vi "GroupRelayControl.vi"(8 "error in (no error)":errorcluster, 9 "Actions":string, 10 "relay names":string, 11 "IVI Refnum in":refnum<k15>) -> (0 "error out":errorcluster, 3 "IVI Refnum out":refnum<k15>)   [LabVIEW 2015]
doc: "Use comma(,) to separate relay names\nExample\nk1,k2,k4\n\nFor action\n20 - Open Relay\n21 - Close Relay\nExample\n20,21,21"
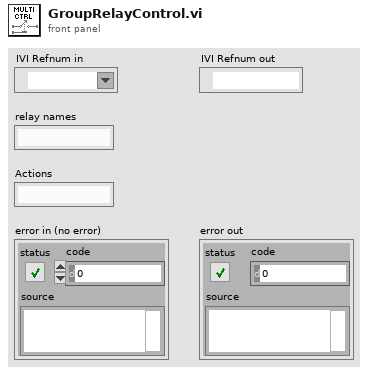
[diagram p1: front panel]
types:
  T1 = typedef "niSwitch Relay Action.ctl" = i32
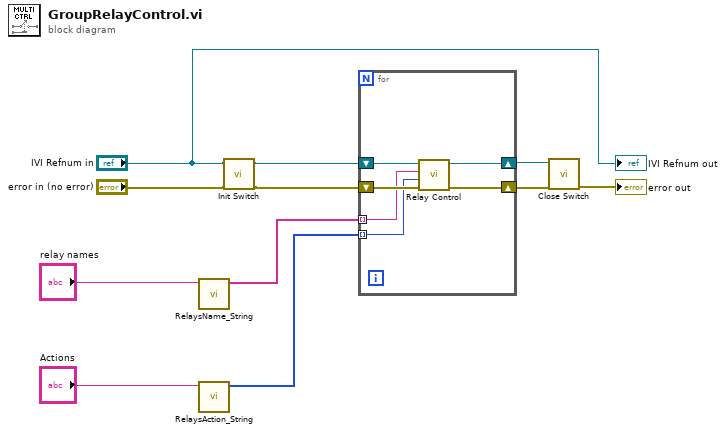
[diagram p0: block diagram]
diagram:
  n1 = call "RelaysName_String.vi"("relay names"="relay names") -> ("Array"=w10:string[])  [unwired: 10 in]
  n2 = call "RelaysAction_String.vi"("Actions"="Actions") -> ("array"=w11:T1[])  [unwired: 10 in]
  n3 = call "Init Switch.vi"("error in (no error)"="error in (no error)", "resource name"="IVI Refnum in") -> ("error out"=w4:errorcluster, "instrument handle out"=w7:refnum<k15>)  [unwired: 8 in]
  n4 = for {
    shift-right: [w15] -> w2
    shift-left: w4 -> [w17]
    shift-right: [w14] -> w3
    shift-left: w7 -> [w16]
    tunnel: w10 -> [w13] mode=indexing
    tunnel: w11 -> [w12] mode=indexing
    n5 = call "Relay Control.vi"("error in (no error)"=w17, "relay action (Close Relay)"=w12, "relay names"=w13, "instrument handle"=w16) -> ("error out"=w15:errorcluster, "instrument handle out"=w14:refnum<k15>)  [unwired: 6 in]
  }
  n6 = call "Close Switch.vi"("error in (no error)"=w2, "instrument handle"=w3) -> ("error out"=→"error out":errorcluster)  [unwired: 9 in]
  "IVI Refnum out" <- "IVI Refnum in"
